vi "Deque Objects.vi"(0 "reference in":refnum<class "Logger.lvclass">, 11 "error in (no error)":errorcluster) -> (6 "remaining elements":T1[](array[typedef]), 15 "error out":errorcluster)   [LabVIEW 2019, in "Logger.lvclass"]
uses:
  Logger.lvclass
  ObjData.ctl
  ObjType.ctl
  Logger.lvclass/Logger.ctl
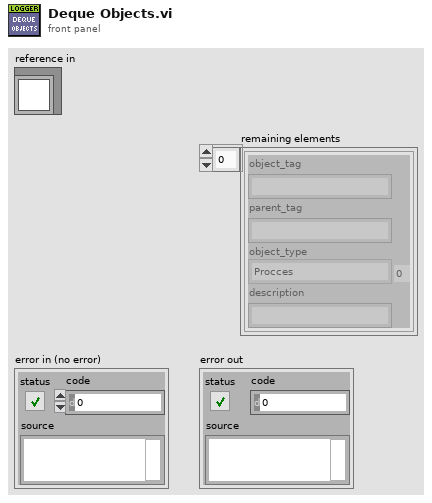
[diagram p1: front panel]
types:
  T1 = typedef "Logger.lvclass/ObjData.ctl" = cluster{"object_tag":string, "parent_tag":string, "object_type":T2, "description":string}
  T2 = typedef "Logger.lvclass/ObjType.ctl" = enum16{"Procces", "Device", "Signal", "DI", "DO", "DA", "AI", "AO", "AA"}
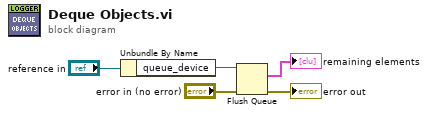
[diagram p0: block diagram]
diagram:
  n1 = Unbundle By Name("reference in") -> ("queue_device"=w2:refnum<queue>)
  n2 = Flush Queue(queue=w2, error in (no error)="error in (no error)") -> (remaining elements=→"remaining elements":T1[], error out=→"error out":errorcluster)  [unwired: 1 out]
